vi "PH_ImageCalibrator.set Source.vi"(0 "i ref in":refnum<vi>, 2 "Source":string, 5 "error in (no error)":errorcluster) -> (14 "i ref out":refnum<vi>, 19 "error out":errorcluster)   [LabVIEW 2014, in "PH_ImageCalibrator.lvlib"]
doc: "This VI checks whther \"Source\" (the cam to deal with) is in the list; if so, the source is set to own attributes."
uses:
  PH_ImageCalibrator.lvlib
  PH_Img_BaseClass/PH_Img_BaseClass.lvlib
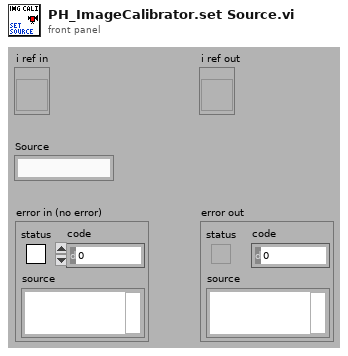
[diagram p1: front panel]
types:
  T1 = typedef "PH_ImageCalibrator.lvlib/PH_ImageCalibrator.i attribute.ctl" = cluster{"GUI Refs":cluster{"Available Cams":refnum<vi>, "OK":refnum<vi>, "Skip":refnum<vi>, "Repeat":refnum<vi>, "Cancel":refnum<vi>, "Length [mm]":refnum<vi>, "Energy [mJ]":refnum<vi>, "Dialog":refnum<vi>}, "Cam instances":string[], "Dark Pics":cluster{"#":i32, "BI taken":bool}, "Lin Cali":cluster{"Distance [Pixel]":dbl, "Distance [mm]":dbl, "Lin Cali Factor [mm/Pixel]":dbl}, "Energy Cali":cluster{"Pixelsum":dbl, "Energy [mJ]":dbl, "Energy Cali factor [mJ/Pixelsum]":dbl, "Underground subtracted?":bool, "#":i32}, "Images":cluster{"Background":T2, "Energy":T2}}
  T2 = typedef "IMAQ Image.ctl" = refnum<image>
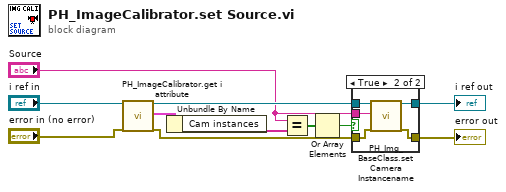
[diagram p0: block diagram]
diagram:
  n1 = call "PH_ImageCalibrator.get i attribute.vi"("i ref in"="i ref in", "error in (no error)"="error in (no error)") -> ("i ref out"=w6:refnum<vi>, "i attribute"=w11:T1, "error out"=w9:errorcluster)  [unwired: 15 in]
  n2 = Unbundle By Name(w11) -> ("Cam instances"=w1:string[])
  n3 = Equal?(x="Source", y=w1) -> (x = y?=w4:bool[])
  n4 = Or Array Elements(Boolean array=w4) -> (logical OR=w3:bool)
  n5 = case shown="True" w3 {
    tunnel: [w13 w18] -> w7
    tunnel: w9 -> [w12 w17]
    tunnel: [w12 w16] -> w10
    tunnel: w6 -> [w13 w15]
    tunnel: "Source" -> [_ w14]
    frame False {
    }
    frame True {
      n6 = call "PH_Img_BaseClass.set Camera Instancename.vi"("i ref in"=w15, "Camera Instancename"=w14, "error in (no error)"=w17) -> ("i ref out"=w18:refnum<vi>, "error out"=w16:errorcluster)  [unwired: 15 in]
    }
  }
  "error out" <- w10
  "i ref out" <- w7
